vi "Add Notes.vi"(8 "error in (no error)":errorcluster, 10 "file events":refnum<class "midi-file-event.lvclass">[](array[class]), 11 "midi-ui in":refnum<class "midi-ui.lvclass">) -> (0 "error out":errorcluster, 3 "midi-ui out":refnum<class "midi-ui.lvclass">)   [LabVIEW 2020, in "midi-ui.lvclass"]
uses:
  midi-ui.lvclass
  midi-file-events/midi-file-event.lvclass
  midi-ui.lvclass/midi-ui.ctl
  midi-file-event.midi/midi-file-event.midi.lvclass
  C:/code/LabVIEW-MIDI/lv-src/midi-file-events/midi-file-event.lvclass
  midi-file-events/midi-file-event.lvclass/midi-file-event.ctl
  midi-file-event.midi/midi-file-event.midi.lvclass/midi-file-event.midi.ctl
  midi-file-events/Delta Tiime.get.vi
  midi-file-event.midi/MIDI_Messages.get.vi
  midi-file-event.midi/Data1.get.vi
  midi-file-event.midi/Data2.get.vi
  midi-file-events/uid.get.vi
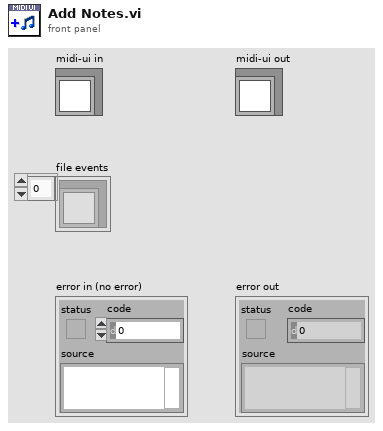
[diagram p1: front panel]
types:
  T1 = map{i32, cluster{"Note On":picture, "Note Off":picture}}
  T2 = map{enum8{"C-2", "C#-2", "D-2", "D#-2", "E-2", "F-2", "F#-2", "G-2", "G#-2", "A-2", "A#-2", "B-2", "C-1", "C#-1", "D-1", "D#-1", "E-1", "F-1", "F#-1", "G-1", "G#-1", "A-1", "A#-1", "B-1", "C0", "C#0", "D0", "D#0", "E0", "F0", "F#0", "G0", "G#0", "A0", "A#0", "B0", "C1", "C#1", "D1", "D#1", "E1", "F1", "F#1", "G1", "G#1", "A1", "A#1", "B1", "C2", "C#2", "D2", "D#2", "E2", "F2", "F#2", "G2", "G#2", "A2", "A#2", "B2", "C3", "C#3", "D3", "D#3", "E3", "F3", "F#3", "G3", "G#3", "A3", "A#3", "B3", "C4", "C#4", "D4", "D#4", "E4", "F4", "F#4", "G4", "G#4", "A4", "A#4", "B4", "C5", "C#5", "D5", "D#5", "E5", "F5", "F#5", "G5", "G#5", "A5", "A#5", "B5", "C6", "C#6", "D6", "D#6", "E6", "F6", "F#6", "G6", "G#6", "A6", "A#6", "B6", "C7", "C#7", "D7", "D#7", "E7", "F7", "F#7", "G7", "G#7", "A7", "A#7", "B7", "C8", "C#8", "D8", "D#8", "E8", "F8", "F#8", "G"}, cluster{"Note Value":enum8{"C-2", "C#-2", "D-2", "D#-2", "E-2", "F-2", "F#-2", "G-2", "G#-2", "A-2", "A#-2", "B-2", "C-1", "C#-1", "D-1", "D#-1", "E-1", "F-1", "F#-1", "G-1", "G#-1", "A-1", "A#-1", "B-1", "C0", "C#0", "D0", "D#0", "E0", "F0", "F#0", "G0", "G#0", "A0", "A#0", "B0", "C1", "C#1", "D1", "D#1", "E1", "F1", "F#1", "G1", "G#1", "A1", "A#1", "B1", "C2", "C#2", "D2", "D#2", "E2", "F2", "F#2", "G2", "G#2", "A2", "A#2", "B2", "C3", "C#3", "D3", "D#3", "E3", "F3", "F#3", "G3", "G#3", "A3", "A#3", "B3", "C4", "C#4", "D4", "D#4", "E4", "F4", "F#4", "G4", "G#4", "A4", "A#4", "B4", "C5", "C#5", "D5", "D#5", "E5", "F5", "F#5", "G5", "G#5", "A5", "A#5", "B5", "C6", "C#6", "D6", "D#6", "E6", "F6", "F#6", "G6", "G#6", "A6", "A#6", "B6", "C7", "C#7", "D7", "D#7", "E7", "F7", "F#7", "G7", "G#7", "A7", "A#7", "B7", "C8", "C#8", "D8", "D#8", "E8", "F8", "F#8", "G"}, "End Time":u32, "Start Time":u32, "on uid":string, "off uid":string}}
  T3 = typedef "midi-ui.lvclass/privatedata.ctl" = cluster{"White Key Length":dbl, "White Key Width":dbl, "Black Key Length":dbl, "Polygon Corners by Name":map{string, cluster{"x":dbl, "y":dbl}[]}, "Anticlockwise rotations [0-3] (0)":i32, "Polygon Corners by Note Name":map{string, cluster{"x":dbl, "y":dbl}[]}, "Picture Control":refnum<vi>, "Owning VI":refnum<vi>, "Control Index":i32, "Note Bounds by Note Name":map{string, cluster{"max":dbl, "min":dbl}}, "Notes on screen":cluster{"Note Value":enum8{"C-2", "C#-2", "D-2", "D#-2", "E-2", "F-2", "F#-2", "G-2", "G#-2", "A-2", "A#-2", "B-2", "C-1", "C#-1", "D-1", "D#-1", "E-1", "F-1", "F#-1", "G-1", "G#-1", "A-1", "A#-1", "B-1", "C0", "C#0", "D0", "D#0", "E0", "F0", "F#0", "G0", "G#0", "A0", "A#0", "B0", "C1", "C#1", "D1", "D#1", "E1", "F1", "F#1", "G1", "G#1", "A1", "A#1", "B1", "C2", "C#2", "D2", "D#2", "E2", "F2", "F#2", "G2", "G#2", "A2", "A#2", "B2", "C3", "C#3", "D3", "D#3", "E3", "F3", "F#3", "G3", "G#3", "A3", "A#3", "B3", "C4", "C#4", "D4", "D#4", "E4", "F4", "F#4", "G4", "G#4", "A4", "A#4", "B4", "C5", "C#5", "D5", "D#5", "E5", "F5", "F#5", "G5", "G#5", "A5", "A#5", "B5", "C6", "C#6", "D6", "D#6", "E6", "F6", "F#6", "G6", "G#6", "A6", "A#6", "B6", "C7", "C#7", "D7", "D#7", "E7", "F7", "F#7", "G7", "G#7", "A7", "A#7", "B7", "C8", "C#8", "D8", "D#8", "E8", "F8", "F#8", "G"}, "End Time":u32, "Start Time":u32}[], "Polygon Pictures by Note Name":map{i32, cluster{"Note On":picture, "Note Off":picture}}, "keyboard":picture[], "Keyboard Note Index by Name":map{i32, i32}, "music":picture[]}
  T4 = cluster{"Note Value":enum8{"C-2", "C#-2", "D-2", "D#-2", "E-2", "F-2", "F#-2", "G-2", "G#-2", "A-2", "A#-2", "B-2", "C-1", "C#-1", "D-1", "D#-1", "E-1", "F-1", "F#-1", "G-1", "G#-1", "A-1", "A#-1", "B-1", "C0", "C#0", "D0", "D#0", "E0", "F0", "F#0", "G0", "G#0", "A0", "A#0", "B0", "C1", "C#1", "D1", "D#1", "E1", "F1", "F#1", "G1", "G#1", "A1", "A#1", "B1", "C2", "C#2", "D2", "D#2", "E2", "F2", "F#2", "G2", "G#2", "A2", "A#2", "B2", "C3", "C#3", "D3", "D#3", "E3", "F3", "F#3", "G3", "G#3", "A3", "A#3", "B3", "C4", "C#4", "D4", "D#4", "E4", "F4", "F#4", "G4", "G#4", "A4", "A#4", "B4", "C5", "C#5", "D5", "D#5", "E5", "F5", "F#5", "G5", "G#5", "A5", "A#5", "B5", "C6", "C#6", "D6", "D#6", "E6", "F6", "F#6", "G6", "G#6", "A6", "A#6", "B6", "C7", "C#7", "D7", "D#7", "E7", "F7", "F#7", "G7", "G#7", "A7", "A#7", "B7", "C8", "C#8", "D8", "D#8", "E8", "F8", "F#8", "G"}, "End Time":u32, "Start Time":u32, "on uid":string, "off uid":string}
  T5 = typedef "midi-file.lvclass/MIDI Messages.ctl" = enum8{"0(0x00)_UnassignedMidiMessage", "1(0x01)_UnassignedMidiMessage", "2(0x02)_UnassignedMidiMessage", "3(0x03)_UnassignedMidiMessage", "4(0x04)_UnassignedMidiMessage", "5(0x05)_UnassignedMidiMessage", "6(0x06)_UnassignedMidiMessage", "7(0x07)_UnassignedMidiMessage", "8(0x08)_NoteOffEvent", "9(0x09)_NoteOnEvent", "10(0x0A)_PolyphonicKeyPressure", "11(0x0B)_ControlChange", "12(0x0C)_ProgramChange", "13(0x0D)_ChannelPressure", "14(0x0E)_PitchBendChange", "15(0x0F)_SystemExclusive(SysEx)", "16(0x10)_UnassignedMidiMessage", "17(0x11)_UnassignedMidiMessage", "18(0x12)_UnassignedMidiMessage", "19(0x13)_UnassignedMidiMessage", "20(0x14)_UnassignedMidiMessage", "21(0x15)_UnassignedMidiMessage", "22(0x16)_UnassignedMidiMessage", "23(0x17)_UnassignedMidiMessage", "24(0x18)_UnassignedMidiMessage", "25(0x19)_UnassignedMidiMessage", "26(0x1A)_UnassignedMidiMessage", "27(0x1B)_UnassignedMidiMessage", "28(0x1C)_UnassignedMidiMessage", "29(0x1D)_UnassignedMidiMessage", "30(0x1E)_UnassignedMidiMessage", "31(0x1F)_UnassignedMidiMessage", "32(0x20)_UnassignedMidiMessage", "33(0x21)_UnassignedMidiMessage", "34(0x22)_UnassignedMidiMessage", "35(0x23)_UnassignedMidiMessage", "36(0x24)_UnassignedMidiMessage", "37(0x25)_UnassignedMidiMessage", "38(0x26)_UnassignedMidiMessage", "39(0x27)_UnassignedMidiMessage", "40(0x28)_UnassignedMidiMessage", "41(0x29)_UnassignedMidiMessage", "42(0x2A)_UnassignedMidiMessage", "43(0x2B)_UnassignedMidiMessage", "44(0x2C)_UnassignedMidiMessage", "45(0x2D)_UnassignedMidiMessage", "46(0x2E)_UnassignedMidiMessage", "47(0x2F)_UnassignedMidiMessage", "48(0x30)_UnassignedMidiMessage", "49(0x31)_UnassignedMidiMessage", "50(0x32)_UnassignedMidiMessage", "51(0x33)_UnassignedMidiMessage", "52(0x34)_UnassignedMidiMessage", "53(0x35)_UnassignedMidiMessage", "54(0x36)_UnassignedMidiMessage", "55(0x37)_UnassignedMidiMessage", "56(0x38)_UnassignedMidiMessage", "57(0x39)_UnassignedMidiMessage", "58(0x3A)_UnassignedMidiMessage", "59(0x3B)_UnassignedMidiMessage", "60(0x3C)_UnassignedMidiMessage", "61(0x3D)_UnassignedMidiMessage", "62(0x3E)_UnassignedMidiMessage", "63(0x3F)_UnassignedMidiMessage", "64(0x40)_UnassignedMidiMessage", "65(0x41)_UnassignedMidiMessage", "66(0x42)_UnassignedMidiMessage", "67(0x43)_UnassignedMidiMessage", "68(0x44)_UnassignedMidiMessage", "69(0x45)_UnassignedMidiMessage", "70(0x46)_UnassignedMidiMessage", "71(0x47)_UnassignedMidiMessage", "72(0x48)_UnassignedMidiMessage", "73(0x49)_UnassignedMidiMessage", "74(0x4A)_UnassignedMidiMessage", "75(0x4B)_UnassignedMidiMessage", "76(0x4C)_UnassignedMidiMessage", "77(0x4D)_UnassignedMidiMessage", "78(0x4E)_UnassignedMidiMessage", "79(0x4F)_UnassignedMidiMessage", "80(0x50)_UnassignedMidiMessage", "81(0x51)_UnassignedMidiMessage", "82(0x52)_UnassignedMidiMessage", "83(0x53)_UnassignedMidiMessage", "84(0x54)_UnassignedMidiMessage", "85(0x55)_UnassignedMidiMessage", "86(0x56)_UnassignedMidiMessage", "87(0x57)_UnassignedMidiMessage", "88(0x58)_UnassignedMidiMessage", "89(0x59)_UnassignedMidiMessage", "90(0x5A)_UnassignedMidiMessage", "91(0x5B)_UnassignedMidiMessage", "92(0x5C)_UnassignedMidiMessage", "93(0x5D)_UnassignedMidiMessage", "94(0x5E)_UnassignedMidiMessage", "95(0x5F)_UnassignedMidiMessage", "96(0x60)_UnassignedMidiMessage", "97(0x61)_UnassignedMidiMessage", "98(0x62)_UnassignedMidiMessage", "99(0x63)_UnassignedMidiMessage", "100(0x64)_UnassignedMidiMessage", "101(0x65)_UnassignedMidiMessage", "102(0x66)_UnassignedMidiMessage", "103(0x67)_UnassignedMidiMessage", "104(0x68)_UnassignedMidiMessage", "105(0x69)_UnassignedMidiMessage", "106(0x6A)_UnassignedMidiMessage", "107(0x6B)_UnassignedMidiMessage", "108(0x6C)_UnassignedMidiMessage", "109(0x6D)_UnassignedMidiMessage", "110(0x6E)_UnassignedMidiMessage", "111(0x6F)_UnassignedMidiMessage", "112(0x70)_UnassignedMidiMessage", "113(0x71)_UnassignedMidiMessage", "114(0x72)_UnassignedMidiMessage", "115(0x73)_UnassignedMidiMessage", "116(0x74)_UnassignedMidiMessage", "117(0x75)_UnassignedMidiMessage", "118(0x76)_UnassignedMidiMessage", "119(0x77)_UnassignedMidiMessage", "120(0x78)_UnassignedMidiMessage", "121(0x79)_UnassignedMidiMessage", "122(0x7A)_UnassignedMidiMessage", "123(0x7B)_UnassignedMidiMessage", "124(0x7C)_UnassignedMidiMessage", "125(0x7D)_UnassignedMidiMessage", "126(0x7E)_UnassignedMidiMessage", "127(0x7F)_UnassignedMidiMessage"}
  T6 = cluster{"left":i16, "top":i16, "right":i16, "bottom":i16}
  T7 = enum8{"C-2", "C#-2", "D-2", "D#-2", "E-2", "F-2", "F#-2", "G-2", "G#-2", "A-2", "A#-2", "B-2", "C-1", "C#-1", "D-1", "D#-1", "E-1", "F-1", "F#-1", "G-1", "G#-1", "A-1", "A#-1", "B-1", "C0", "C#0", "D0", "D#0", "E0", "F0", "F#0", "G0", "G#0", "A0", "A#0", "B0", "C1", "C#1", "D1", "D#1", "E1", "F1", "F#1", "G1", "G#1", "A1", "A#1", "B1", "C2", "C#2", "D2", "D#2", "E2", "F2", "F#2", "G2", "G#2", "A2", "A#2", "B2", "C3", "C#3", "D3", "D#3", "E3", "F3", "F#3", "G3", "G#3", "A3", "A#3", "B3", "C4", "C#4", "D4", "D#4", "E4", "F4", "F#4", "G4", "G#4", "A4", "A#4", "B4", "C5", "C#5", "D5", "D#5", "E5", "F5", "F#5", "G5", "G#5", "A5", "A#5", "B5", "C6", "C#6", "D6", "D#6", "E6", "F6", "F#6", "G6", "G#6", "A6", "A#6", "B6", "C7", "C#7", "D7", "D#7", "E7", "F7", "F#7", "G7", "G#7", "A7", "A#7", "B7", "C8", "C#8", "D8", "D#8", "E8", "F8", "F#8", "G"}
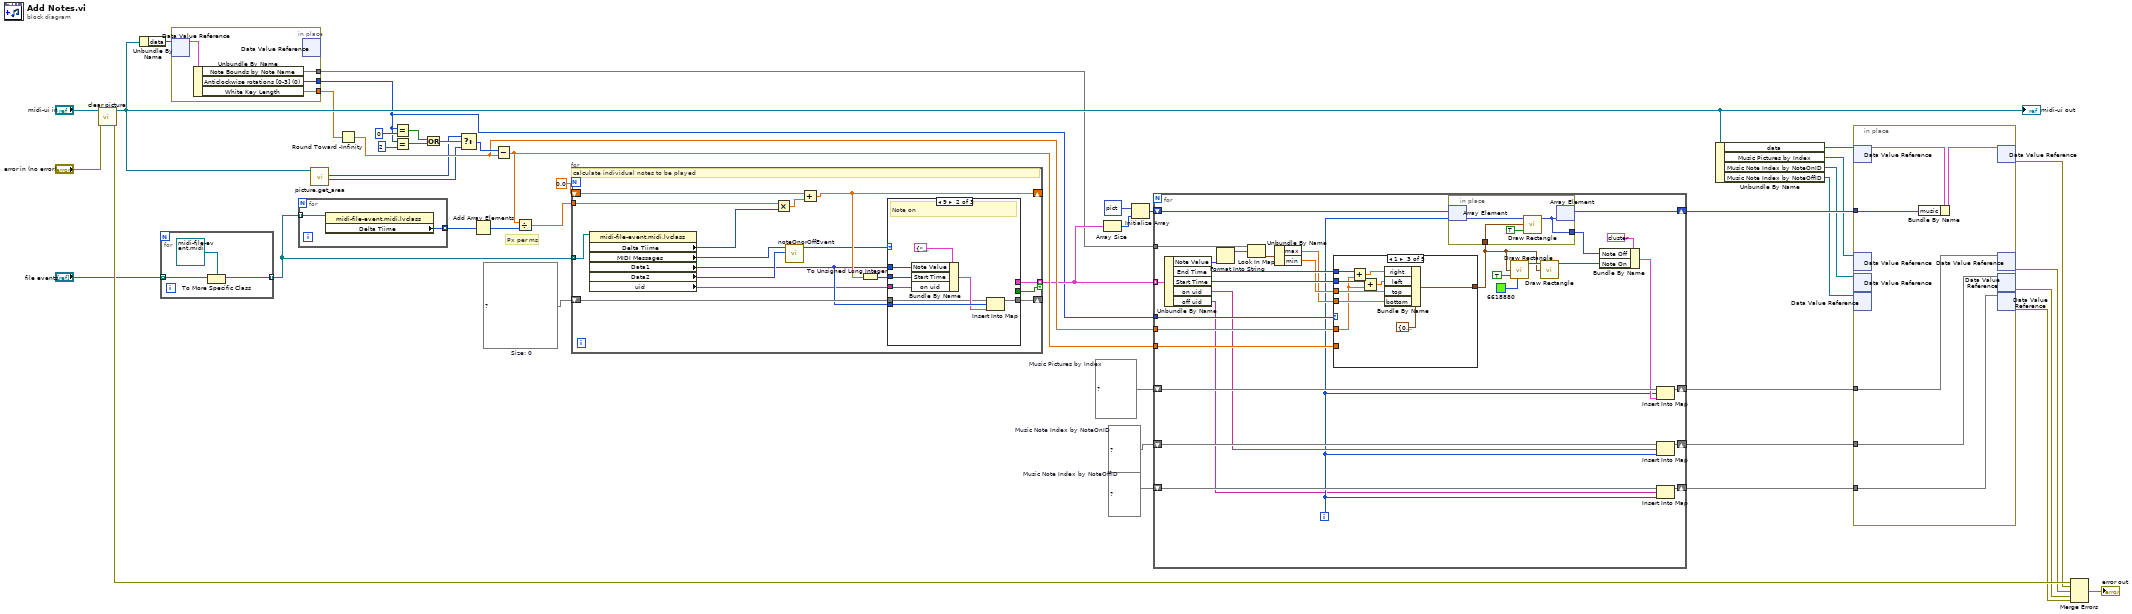
[diagram p0: block diagram]
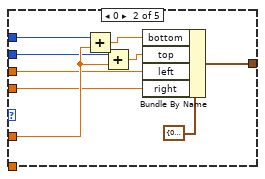
[diagram p3: hidden frame]
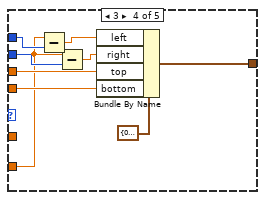
[diagram p4: hidden frame]
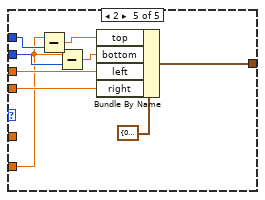
[diagram p5: hidden frame]
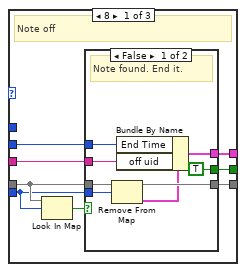
[diagram p6: hidden frame]
diagram:
  w24 = map{string, i32} {}  # Music Note Index by NoteOffID
  w29 = T1 {}  # Music Pictures by Index
  w30 = map{string, i32} {}  # Music Note Index by NoteOnID
  w36 = T2 {}  # Size: 0
  # "Px per ms"
  n1 = call "clear picture.vi"("error in"="error in (no error)", "midi-ui in"="midi-ui in") -> ("error out"=w8:errorcluster, "midi-ui out"=w19:refnum<class "midi-ui.lvclass">)  [unwired: 8 in]
  "midi-ui out" <- w19
  n2 = Unbundle By Name(w19) -> ("data"=w18:refnum<data-value>)
  n3 = for {
    tunnel: "file events" -> [w48] mode=indexing
    tunnel: [w46] -> w1 mode=indexing
    n4 = To More Specific Class(target class=refnum<class "midi-file-event.midi.lvclass"> refnum ("midi-file-event.midi.lvclass"), reference=w48) -> (specific class reference=w46:refnum<class "midi-file-event.midi.lvclass">)  [unwired: 1 in, 1 out]
  }
  n5 = in-place {
    in-place-border: [w51] -> w17
    in-place-border: [w50] -> w16
    in-place-border: [w49] -> w15
    n6 = in-place-dvr #1(w18) -> (w52:T3)  [unwired: 1 out]
    n7 = Unbundle By Name(w52) -> ("Note Bounds by Note Name"=w49:map{string, cluster{"max":dbl, "min":dbl}}, "Anticlockwise rotations [0-3] (0)"=w51:i32, "White Key Length"=w50:dbl)
    n8 = in-place-dvr #1() -> ()  [unwired: 1 in, 2 out]
  }
  n9 = for {
    tunnel: w1 -> [w54] mode=indexing
    tunnel: [w53] -> w45 mode=indexing
    n10 = property class="midi-file-event.midi.lvclass"(reference=w54) -> ("Delta Tiime"=w53:u32)  [unwired: 1 in, 2 out]
  }
  n11 = call "picture.get_area.vi"("midi-ui in"=w19) -> ("Bounds:Area Width"=w20:u32, "Bounds:Area Height"=w21:u32)  [unwired: 7 in, 2 out]
  n12 = Round Toward -Infinity(1:w16) -> (0:w34:dbl)
  n13 = Equal?(x=w17, y=0) -> (x = y?=w42:bool)
  n14 = Equal?(x=w17, y=2) -> (x = y?=w41:bool)
  n15 = Or(x=w42, y=w41) -> (x .or. y?=w40:bool)
  n16 = Select(t=w21, s=w40, f=w20) -> (s? t:f=w39:u32)
  n17 = Add Array Elements(numeric array=w45) -> (sum=w38:u32)
  n18 = Subtract(x=w39, y=w34) -> (x-y=w33:dbl)
  n19 = Divide(x=w33, y=w38) -> (x/y=w37:dbl)
  n20 = for {
    tunnel: w1 -> [w60] mode=indexing
    shift-right: [w67] -> _
    shift-left: 0.0 -> [w70]
    shift-right: [w68] -> _
    shift-left: w36 -> [w69]
    tunnel: [w66] -> w28 mode=indexing if=w65
    tunnel: w37 -> [w63]
    # "calculate individual notes to be played"
    n21 = property class="midi-file-event.midi.lvclass"(reference=w60) -> ("Delta Tiime"=w59:u32, "MIDI Messages"=w58:T5, "Data1"=w56:u8, "Data2"=w57:u8, "uid"=w55:string)  [unwired: 1 in, 2 out]
    n22 = Multiply(x=w63, y=w59) -> (x*y=w64:dbl)
    n23 = call "noteOnorOffEvent.vi"("Volume"=w57, "MIDI Message"=w58) -> ("Midi Message"=w62:u16)  [unwired: 9 in]
    n24 = Add(x=w70, y=w64) -> (x+y=w67:dbl)
    n25 = To Unsigned Long Integer(number=w67) -> (unsigned 32bit integer=w61:u32)
    n26 = case shown="9" w62 {
      tunnel: w69 -> [w74 w89 w96]
      tunnel: w56 -> [w73 w95 _]
      tunnel: [w78 w92 w96] -> w68
      tunnel: w56 -> [_ w94 _]
      tunnel: w61 -> [w77 w93 _]
      tunnel: [w76 _ _] -> w66
      tunnel: [w75 _ _] -> w65
      tunnel: w55 -> [w71 w90 _]
      frame 8 {
        # "Note off"
        n27 = Look In Map(map=w74, key=w73) -> (key not found?=w72:bool)  [unwired: 1 in, 1 out]
        n28 = case shown="False" w72 {
          tunnel: [w82 w87] -> w78
          tunnel: w74 -> [w83 w87]
          tunnel: w77 -> [w86 _]
          tunnel: [w85 _] -> w76
          tunnel: [TRUE _] -> w75
          tunnel: w73 -> [w81 _]
          tunnel: w71 -> [w79 _]
          frame False {
            # "Note found. End it."
            n29 = Remove From Map(10:w81, 11:w83) -> (1:w80:T4, 3:w82:T2)  [unwired: 1 out]
            n30 = Bundle By Name(cluster=w80, "End Time"=w86, "off uid"=w79) -> (w85:T4)
          }
          frame True {
            # "Not found so ignore"
          }
        }
      }
      frame 9 {
        # "Note on"
        n31 = Bundle By Name(cluster=T4 {"Note Value"=enum."C-2", "End Time"=0, "Start Time"=0, "on uid"="", "off uid"=""}, "Note Value"=w94, "Start Time"=w93, "on uid"=w90) -> (w91:T4)
        n32 = Insert Into Map(map in=w89, key=w95, value=w91) -> (map out=w92:T2)  [unwired: 2 out]
      }
      frame Default {
      }
    }
  }
  n33 = Array Size(array=w28) -> (size(s)=w27:i32)
  n34 = Initialize Array(picture data[5B] ("picture"), w27) -> (w25:picture[])
  n35 = for {
    tunnel: w28 -> [w127] mode=indexing
    tunnel: w15 -> [w124]
    tunnel: w17 -> [w119]
    tunnel: w34 -> [w118]
    tunnel: w33 -> [w117]
    shift-right: [w113] -> w9
    shift-left: w29 -> [w114]
    shift-right: [w112] -> w10
    shift-left: w30 -> [w116]
    shift-right: [w102] -> w22
    shift-left: w25 -> [w103]
    shift-right: [w100] -> w11
    shift-left: w24 -> [w101]
    i -> [w99]
    n36 = Unbundle By Name(w127) -> ("Note Value"=w122:T7, "End Time"=w125:u32, "Start Time"=w126:u32, "on uid"=w104:string, "off uid"=w98:string)
    n37 = Format Into String(w122) -> (resulting string=w115:string)  [unwired: 3 in, 1 out]
    n38 = Look In Map(map=w124, key=w115) -> (value=w123:cluster{"max":dbl, "min":dbl})  [unwired: 1 in, 1 out]
    n39 = Unbundle By Name(w123) -> ("max"=w120:dbl, "min"=w121:dbl)
    n40 = case shown="1" w119 {
      tunnel: w126 -> [_ w135 w144 w153 w162]
      tunnel: w125 -> [_ w137 w145 w154 w163]
      tunnel: [_ w132 w148 w157 w166] -> w107
      tunnel: w121 -> [_ w134 w147 w156 w165]
      tunnel: w120 -> [_ w133 w146 w155 w164]
      tunnel: w118 -> [_ w136 w141 _ _]
      tunnel: w117 -> [_ _ _ w150 w159]
      frame Default {
      }
      frame 0 {
        n41 = Add(x=w137, y=w136) -> (x+y=w139:dbl)
        n42 = Add(x=w135, y=w136) -> (x+y=w138:dbl)
        n43 = Bundle By Name(cluster=T6 {"left"=0, "top"=0, "right"=0, "bottom"=0} ("rect"), "bottom"=w139, "top"=w138, "left"=w134, "right"=w133) -> (w132:T6)
      }
      frame 1 {
        n44 = Add(x=w145, y=w141) -> (x+y=w143:dbl)
        n45 = Add(x=w144, y=w141) -> (x+y=w142:dbl)
        n46 = Bundle By Name(cluster=T6 {"left"=0, "top"=0, "right"=0, "bottom"=0} ("rect"), "right"=w143, "left"=w142, "top"=w147, "bottom"=w146) -> (w148:T6)
      }
      frame 3 {
        n47 = Subtract(x=w150, y=w154) -> (x-y=w152:dbl)
        n48 = Subtract(x=w150, y=w153) -> (x-y=w151:dbl)
        n49 = Bundle By Name(cluster=T6 {"left"=0, "top"=0, "right"=0, "bottom"=0} ("rect"), "left"=w152, "right"=w151, "top"=w156, "bottom"=w155) -> (w157:T6)
      }
      frame 2 {
        n50 = Subtract(x=w159, y=w163) -> (x-y=w161:dbl)
        n51 = Subtract(x=w159, y=w162) -> (x-y=w160:dbl)
        n52 = Bundle By Name(cluster=T6 {"left"=0, "top"=0, "right"=0, "bottom"=0} ("rect"), "top"=w161, "bottom"=w160, "left"=w165, "right"=w164) -> (w166:T6)
      }
    }
    n53 = in-place {
      in-place-border: w107 -> [w130]
      in-place-border: [w129] -> w97
      n54 = in-place-array #2(w103, w99) -> (w128:picture)
      n55 = call <vilib>:"Draw Rectangle.vi"("picture"=w128, "rect"=w130, "fill?(F)"=TRUE) -> ("new picture"=w129:picture)  [unwired: 6 in]
      n56 = in-place-array #2(w129) -> (w102:picture[])  [unwired: 1 out]
    }
    n57 = call <vilib>:"Draw Rectangle.vi"("rect"=w107, "fill?(F)"=TRUE, "color(black)"=u32 6618880) -> ("new picture"=w108:picture)  [unwired: 6 in]
    n58 = call <vilib>:"Draw Rectangle.vi"("picture"=w108, "rect"=w107) -> ("new picture"=w106:picture)  [unwired: 7 in]
    n59 = Bundle By Name(cluster=cluster{"Note On":picture, "Note Off":picture} {"Note On"=bytes[0], "Note Off"=bytes[0]} ("value"), "Note Off"=w97, "Note On"=w106) -> (w105:cluster{"Note On":picture, "Note Off":picture})
    n60 = Insert Into Map(map in=w114, key=w99, value=w105) -> (map out=w113:T1)  [unwired: 2 out]
    n61 = Insert Into Map(map in=w116, key=w104, value=w99) -> (map out=w112:map{string, i32})  [unwired: 2 out]
    n62 = Insert Into Map(map in=w101, key=w98, value=w99) -> (map out=w100:map{string, i32})  [unwired: 2 out]
  }
  n63 = Unbundle By Name(w19) -> ("data"=w23:refnum<data-value>, "Music Pictures by Index"=w14:refnum<data-value>, "Music Note Index by NoteOnID"=w13:refnum<data-value>, "Music Note Index by NoteOffID"=w12:refnum<data-value>)
  n64 = in-place {
    in-place-border: w22 -> [w171]
    in-place-border: w11 -> [w170]
    in-place-border: w10 -> [w169]
    in-place-border: w9 -> [w168]
    n65 = in-place-dvr #3(w23) -> (w173:T3)  [unwired: 1 out]
    n66 = in-place-dvr #4(w14) -> ()  [unwired: 2 out]
    n67 = in-place-dvr #5(w13) -> ()  [unwired: 2 out]
    n68 = in-place-dvr #6(w12) -> ()  [unwired: 2 out]
    n69 = Bundle By Name(cluster=w173, "music"=w171) -> (w172:T3)
    n70 = in-place-dvr #3(w172) -> (w7:errorcluster)  [unwired: 1 out]
    n71 = in-place-dvr #4(w168) -> (w6:errorcluster)  [unwired: 1 out]
    n72 = in-place-dvr #5(w169) -> (w5:errorcluster)  [unwired: 1 out]
    n73 = in-place-dvr #6(w170) -> (w4:errorcluster)  [unwired: 1 out]
  }
  n74 = Merge Errors(w8, w7, w6, w5, w4) -> (→"error out":errorcluster)
